vi "rsidr_core_global.vi"() -> ()   [LabVIEW 2020, in "Rohde&Schwarz RTx Oscilloscopes.lvlib"] (continued)
Options"="", "Flags"=0, "Help"="Queries the digital probe state.\n\nAvailable Repeated Capabilities:\nDigital: D0, D1, D2, D3, D4, D5, D6, D7, D8, D9, D10, D11, D12, D13, D14, D15\r\n\nRemote-control command(s):\nDIGital<m>:PROBe:ENABle?"}, {"Level"=2, "Class Only"=FALSE, "Identifier"="RSRTX_ATTR_DIGITAL_POINT_SELECTION", "Descriptive Name"="Digital Point Selection", "Data Type"=0, "Command"="DIG{Digital}:DATA:POIN", "Access"=1, "Range Table"="RsRtx_rngPointSelection", "Read Callback"="", "Write Callback"="", "Supported Models"="", "Instrument Options"="", "Flags"=0, "Help"="Selects a range of samples that will be returned. Depending on the current settings, the memory can contain more data samples than the screen is able to display. In this case, you can decide which data will be saved: samples stored in the memory or only the displayed samples.\n\nAvailable Repeated Capabilities:\nDigital: D0, D1, D2, D3, D4, D5, D6, D7, D8, D9, D10, D11, D12, D13, D14, D15\r\n\nRemote-control command(s):\nDIGital<m>:DATA:POINts"}, {"Level"=1, "Class Only"=TRUE, "Identifier"="", "Descriptive Name"="Logic", "Data Type"=0, "Command"="", "Access"=0, "Range Table"="", "Read Callback"="", "Write Callback"="", "Supported Models"="", "Instrument Options"="", "Flags"=0, "Help"="Configures the logic probe."}, {"Level"=2, "Class Only"=FALSE, "Identifier"="RSRTX_ATTR_LOGIC_STATE", "Descriptive Name"="Logic State", "Data Type"=3, "Command"="LOG{Logic}:STAT", "Access"=2, "Range Table"="", "Read Callback"="", "Write Callback"="", "Supported Models"="", "Instrument Options"="", "Flags"=0, "Help"="Enables the logic probe.\n\nAvailable Repeated Capabilities:\nLogic: Logic1, Logic2\r\n\nRemote-control command(s):\nLOGic<p>:STATe"}, {"Level"=2, "Class Only"=FALSE, "Identifier"="RSRTX_ATTR_LOGIC_TYPE", "Descriptive Name"="Logic Type", "Data Type"=0, "Command"="LOG{Logic}:TYPE", "Access"=2, "Range Table"="RsRtx_rngLogicType", "Read Callback"="", "Write Callback"="", "Supported Models"="", "Instrument Options"="", "Flags"=0, "Help"="Selects the logic type.\n\nAvailable Repeated Capabilities:\nLogic: Logic1, Logic2\r\n\nRemote-control command(s):\nLOGic<p>:TYPE"}, {"Level"=2, "Class Only"=FALSE, "Identifier"="RSRTX_ATTR_LOGIC_THRESHOLD", "Descriptive Name"="Logic Threshold", "Data Type"=0, "Command"="LOG{Logic}:THR", "Access"=2, "Range Table"="RsRtx_rngLogicThreshold", "Read Callback"="", "Write Callback"="", "Supported Models"="", "Instrument Options"="", "Flags"=0, "Help"="Configures logic threshold.\n\nAvailable Repeated Capabilities:\nLogic: Logic1, Logic2\r\n\nRemote-control command(s):\nLOGic<p>:THReshold"}, {"Level"=2, "Class Only"=FALSE, "Identifier"="RSRTX_ATTR_LOGIC_THRESHOLD_USER_LEVEL", "Descriptive Name"="Logic Threshold User Level", "Data Type"=1, "Command"="LOG{Logic}:THR:UDL", "Access"=2, "Range Table"="", "Read Callback"="", "Write Callback"="", "Supported Models"="", "Instrument Options"="", "Flags"=0, "Help"="Configures threshold user level.\n\nAvailable Repeated Capabilities:\nLogic: Logic1, Logic2\r\n\nRemote-control command(s):\nLOGic<p>:THReshold:UDLevel"}, {"Level"=2, "Class Only"=FALSE, "Identifier"="RSRTX_ATTR_LOGIC_HYSTERESIS", "Descriptive Name"="Logic Hysteresis", "Data Type"=0, "Command"="LOG{Logic}:HYST", "Access"=2, "Range Table"="rsrtx_rngLogicHysteresis", "Read Callback"="", "Write Callback"="", "Supported Models"="", "Instrument Options"="", "Flags"=0, "Help"="Configures logic hysteresis.\n\nAvailable Repeated Capabilities:\nLogic: Logic1, Logic2\r\n\nRemote-control command(s):\nLOGic<p>:HYSTeresis"}, {"Level"=2, "Class Only"=FALSE, "Identifier"="RSRTX_ATTR_LOGIC_ARITHMETICS", "Descriptive Name"="Logic Arithmetics", "Data Type"=0, "Command"="LOG{Logic}:ARIT", "Access"=2, "Range Table"="rsrtx_rngWaveformArithmetics", "Read Callback"="", "Write Callback"="", "Supported Models"="", "Instrument Options"="", "Flags"=0, "Help"="Configures logic arithmetics.\n\nAvailable Repeated Capabilities:\nLogic: Logic1, Logic2\r\n\nRemote-control command(s):\nLOGic<p>:ARIThmetics"}, {"Level"=2, "Class Only"=FALSE, "Identifier"="RSRTX_ATTR_LOGIC_PROBE_CONNECTED", "Descriptive Name"="Logic Probe Connected", "Data Type"=3, "Command"="LOG{Logic}:PROB?", "Access"=0, "Range Table"="", "Read Callback"="", "Write Callback"="", "Supported Models"="", "Instrument Options"="", "Flags"=0, "Help"="Checks if the logic probe is connected.\n\nAvailable Repeated Capabilities:\nLogic: Logic1, Logic2\r\n\nRemote-control command(s):\nLOGic<p>:PROBe[:ENABle]?"}, {"Level"=2, "Class Only"=FALSE, "Identifier"="RSRTX_ATTR_LOGIC_CURRENT_MAXIMUM", "Descriptive Name"="Logic Current Maximum", "Data Type"=0, "Command"="LOG{Logic}:CURR:STAT:MAX?", "Access"=0, "Range Table"="RsRtx_rngLogicCurrent", "Read Callback"="", "Write Callback"="", "Supported Models"="", "Instrument Options"="", "Flags"=0, "Help"="Queries current maximum.\n\nAvailable Repeated Capabilities:\nLogic: Logic1, Logic2\r\n\nRemote-control command(s):\nLOGic<p>:CURRent:STATe:MAXimum?"}, {"Level"=2, "Class Only"=FALSE, "Identifier"="RSRTX_ATTR_LOGIC_CURRENT_MINIMUM", "Descriptive Name"="Logic Current Minimum", "Data Type"=0, "Command"="LOG{Logic}:CURR:STAT:MIN?", "Access"=0, "Range Table"="RsRtx_rngLogicCurrent", "Read Callback"="", "Write Callback"="", "Supported Models"="", "Instrument Options"="", "Flags"=0, "Help"="Queries current minimum.\n\nAvailable Repeated Capabilities:\nLogic: Logic1, Logic2\r\n\nRemote-control command(s):\nLOGic<p>:CURRent:STATe:MINimum?"}, {"Level"=2, "Class Only"=FALSE, "Identifier"="RSRTX_ATTR_LOGIC_POINT_SELECTION", "Descriptive Name"="Logic Point Selection", "Data Type"=0, "Command"="LOG{Logic}:DATA:POIN", "Access"=1, "Range Table"="RsRtx_rngPointSelection", "Read Callback"="", "Write Callback"="", "Supported Models"="", "Instrument Options"="", "Flags"=0, "Help"="Selects a range of samples that will be returned with LOGic<p>:DATA. Depending on the current settings, the memory can contain more data samples than the screen is able to display. In this case, you can decide which data will be saved: samples stored in the memory or only the displayed samples.\n\nNote: The sample range can be changed only in STOP mode. If the acquisition is running, DEF is always used automatically. If the acquisition has been stopped, data can be read from the memory, and all settings are available.\n\nAvailable Repeated Capabilities:\nLogic: Logic1, Logic2\r\n\nRemote-control command(s):\nLOGic<p>:DATA:POINts"}, {"Level"=2, "Class Only"=FALSE, "Identifier"="RSRTX_ATTR_LOGIC_WAVEFORM_DATA_POINTS", "Descriptive Name"="Logic Waveform Data Points", "Data Type"=0, "Command"="LOG{Logic}:DATA:POIN?", "Access"=0, "Range Table"="", "Read Callback"="", "Write Callback"="", "Supported Models"="", "Instrument Options"="", "Flags"=0, "Help"="Returns the number of returned samples for the selected range.\n\nAvailable Repeated Capabilities:\nLogic: Logic1, Logic2\r\n\nRemote-control command(s):\nLOGic<p>:DATA:POINts?"}, {"Level"=1, "Class Only"=TRUE, "Identifier"="", "Descriptive Name"="Triggering Subsystem", "Data Type"=0, "Command"="", "Access"=0, "Range Table"="", "Read Callback"="", "Write Callback"="", "Supported Models"="", "Instrument Options"="", "Flags"=0, "Help"="Attributes that control how the oscilloscope triggers."}, {"Level"=2, "Class Only"=FALSE, "Identifier"="RSRTX_ATTR_TRIGGER_TYPE_A", "Descriptive Name"="Trigger Type A", "Data Type"=0, "Command"="TRIG:A:TYPE", "Access"=2, "Range Table"="rsrtx_rngTriggerType", "Read Callback"="", "Write Callback"="", "Supported Models"="", "Instrument Options"="", "Flags"=0, "Help"="Sets the trigger type.\n\nAvailable Repeated Capabilities:\nNone\n\nRemote-control command(s):\nTRIGger:A:TYPE"}, {"Level"=2, "Class Only"=FALSE, "Identifier"="RSRTX_ATTR_TRIGGER_SOURCE_A", "Descriptive Name"="Trigger Source A", "Data Type"=0, "Command"="TRIG:A:SOUR", "Access"=2, "Range Table"="rsrtx_rngTriggerSource", "Read Callback"="", "Write Callback"="", "Supported Models"="", "Instrument Options"="", "Flags"=0, "Help"="Sets the trigger source for the selected trigger type.\n\nAvailable Repeated Capabilities:\nNone\n\nRemote-control command(s):\nTRIGger:A:SOURce"}, {"Level"=2, "Class Only"=FALSE, "Identifier"="RSRTX_ATTR_TRIGGER_SOURCE_B", "Descriptive Name"="Trigger Source B", "Data Type"=0, "Command"="TRIG:B:SOUR", "Access"=2, "Range Table"="rsrtx_rngTriggerSource", "Read Callback"="", "Write Callback"="", "Supported Models"="", "Instrument Options"="", "Flags"=0, "Help"="Sets the trigger source for the selected trigger type.\n\nAvailable Repeated Capabilities:\nNone\n\nRemote-control command(s):\nTRIGger:B:SOURce"}, {"Level"=2, "Class Only"=FALSE, "Identifier"="RSRTX_ATTR_EXTERNAL_TRIGGER_COUPLING", "Descriptive Name"="External Trigger Coupling", "Data Type"=0, "Command"="TRIG:EXT:COUP", "Access"=2, "Range Table"="rsrtx_rngExternalTriggerCoupling", "Read Callback"="", "Write Callback"="", "Supported Models"="", "Instrument Options"="", "Flags"=0, "Help"="Sets the coupling for the external trigger input.\n\nAvailable Repeated Capabilities:\nNone\n\nRemote-control command(s):\nTRIGger:EXTern:COUPling"}, {"Level"=2, "Class Only"=FALSE, "Identifier"="RSRTX_ATTR_EXTERNAL_TRIGGER_TERMINATION", "Descriptive Name"="External Trigger Termination", "Data Type"=3, "Command"="TRIG:EXT:TERM", "Access"=2, "Range Table"="", "Read Callback"="", "Write Callback"="", "Supported Models"="", "Instrument Options"="", "Flags"=0, "Help"="Adjusts the input impedance of the external trigger input.\nOnly available for instruments with 1 GHz bandwidth.\n\nAvailable Repeated Capabilities:\nNone\n\nRemote-control command(s):\nTRIGger:EXTern:TERMination"}, {"Level"=2, "Class Only"=FALSE, "Identifier"="RSRTX_ATTR_EXTERNAL_TRIGGER_OVERLOAD", "Descriptive Name"="External Trigger Overload", "Data Type"=3, "Command"="TRIG:EXT:OVER", "Access"=2, "Range Table"="", "Read Callback"="", "Write Callback"="", "Supported Models"="", "Instrument Options"="", "Flags"=0, "Help"="Retrieves the overload status of the external trigger input from the status bit. When the overload problem is solved, use the command to reset the status bit.\nOnly available for instruments with 1 GHz bandwidth.\n\nAvailable Repeated Capabilities:\nNone\n\nRemote-control command(s):\nTRIGger:EXTern:OVERload"}, {"Level"=2, "Class Only"=FALSE, "Identifier"="RSRTX_ATTR_TRIGGER_HOLDOFF_TIME", "Descriptive Name"="Trigger Holdoff Time", "Data Type"=1, "Command"="TRIG:A:HOLD:TIME", "Access"=2, "Range Table"="", "Read Callback"="", "Write Callback"="", "Supported Models"="", "Instrument Options"="", "Flags"=0, "Help"="Defines the holdoff time. The next trigger occurs only after the holdoff time has passed.\n\nAvailable Repeated Capabilities:\nNone\n\nRemote-control command(s):\nTRIGger:A:HOLDoff:TIME"}, {"Level"=2, "Class Only"=FALSE, "Identifier"="RSRTX_ATTR_TRIGGER_HOLDOFF_MODE", "Descriptive Name"="Trigger Holdoff Mode", "Data Type"=0, "Command"="TRIG:A:HOLD:MODE", "Access"=2, "Range Table"="rsrtx_rngTriggerHoldoffMode", "Read Callback"="", "Write Callback"="", "Supported Models"="", "Instrument Options"="", "Flags"=0, "Help"="Enables or disables the holdoff time.\n\nAvailable Repeated Capabilities:\nNone\n\nRemote-control command(s):\nTRIGger:A:HOLDoff:MODE"}, {"Level"=2, "Class Only"=FALSE, "Identifier"="RSRTX_ATTR_TRIGGER_HYSTERESIS_A", "Descriptive Name"="Trigger Hysteresis A", "Data Type"=0, "Command"="TRIG:A:HYST", "Access"=2, "Range Table"="rsrtx_rngHysteresisMode", "Read Callback"="", "Write Callback"="", "Supported Models"="", "Instrument Options"="", "Flags"=0, "Help"="Sets a hysteresis range around the trigger level of the A trigger event. If the signal jitters inside this range and crosses the trigger level thereby, no trigger event occurs. Hysteresis is available for edge and width trigger.\n\nAvailable Repeated Capabilities:\nNone\n\nRemote-control command(s):\nTRIGger:A:HYSTeresis"}, {"Level"=2, "Class Only"=FALSE, "Identifier"="RSRTX_ATTR_TRIGGER_HYSTERESIS_A_LEVEL", "Descriptive Name"="Trigger Hysteresis A Level", "Data Type"=0, "Command"="TRIG:A:LEV1:HYST", "Access"=2, "Range Table"="", "Read Callback"="", "Write Callback"="", "Supported Models"="RTM|RTA", "Instrument Options"="", "Flags"=0, "Help"="Sets the hysteresis value if TRIGger:A:HYSTeresis is set to MANual. Only available on instruments with 1 GHz bandwidth.\n\nAvailable Repeated Capabilities:\nNone\n\nRemote-control command(s):\nTRIGger:A:LEVel<n>:HYSTeresis"}, {"Level"=2, "Class Only"=FALSE, "Identifier"="RSRTX_ATTR_TRIGGER_HYSTERESIS_B", "Descriptive Name"="Trigger Hysteresis B", "Data Type"=0, "Command"="TRIG:B:HYST", "Access"=2, "Range Table"="rsrtx_rngHysteresisMode", "Read Callback"="", "Write Callback"="", "Supported Models"="", "Instrument Options"="", "Flags"=0, "Help"="Sets a hysteresis range around the trigger level of the A trigger event. If the signal jitters inside this range and crosses the trigger level thereby, no trigger event occurs. Hysteresis is available for edge and width trigger.\n\nAvailable Repeated Capabilities:\nNone\n\nRemote-control command(s):\nTRIGger:B:HYSTeresis"}, {"Level"=2, "Class Only"=FALSE, "Identifier"="RSRTX_ATTR_TRIGGER_HYSTERESIS_B_LEVEL", "Descriptive Name"="Trigger Hysteresis B Level", "Data Type"=0, "Command"="TRIG:B:LEV:HYST", "Access"=2, "Range Table"="", "Read Callback"="", "Write Callback"="", "Supported Models"="", "Instrument Options"="", "Flags"=0, "Help"="Sets the hysteresis value if TRIGger:B:HYSTeresis is set to MANual. Only available on instruments with 1 GHz bandwidth.\n\nAvailable Repeated Capabilities:\nNone\n\nRemote-control command(s):\nTRIGger:B:LEVel:HYSTeresis"}, {"Level"=2, "Class Only"=FALSE, "Identifier"="RSRTX_ATTR_TRIGGER_ENABLED", "Descriptive Name"="Trigger Enabled", "Data Type"=3, "Command"="TRIG:B:ENAB", "Access"=2, "Range Table"="", "Read Callback"="", "Write Callback"="", "Supported Models"="", "Instrument Options"="", "Flags"=0, "Help"="Activates or deactivates the second trigger. The instrument triggers if both trigger event conditions (A and B) are fulfilled.\n\nAvailable Repeated Capabilities:\nNone\n\nRemote-control command(s):\nTRIGger:B:ENABle"}, {"Level"=2, "Class Only"=FALSE, "Identifier"="RSRTX_ATTR_TRIGGER_MODIFIER_A", "Descriptive Name"="Trigger Modifier A", "Data Type"=0, "Command"="TRIG:A:MODE", "Access"=2, "Range Table"="rsrtx_rngTriggerMode", "Read Callback"="", "Write Callback"="", "Supported Models"="", "Instrument Options"="", "Flags"=0, "Help"="Sets the trigger mode. The trigger mode determines the behaviour of the instrument if no trigger occurs.\n\nAvailable Repeated Capabilities:\nNone\n\nRemote-control command(s):\nTRIGger:A:MODE"}, {"Level"=2, "Class Only"=FALSE, "Identifier"="RSRTX_ATTR_TRIGGER_MODIFIER_B", "Descriptive Name"="Trigger Modifier B", "Data Type"=0, "Command"="TRIG:B:MODE", "Access"=2, "Range Table"="rsrtx_rngTriggerMode", "Read Callback"="", "Write Callback"="", "Supported Models"="", "Instrument Options"="", "Flags"=0, "Help"="Sets the trigger mode. The trigger mode determines the behaviour of the instrument if no trigger occurs.\n\nAvailable Repeated Capabilities:\nNone\n\nRemote-control command(s):\nTRIGger:B:MODE"}, {"Level"=2, "Class Only"=FALSE, "Identifier"="RSRTX_ATTR_TRIGGER_EVENT_COUNT", "Descriptive Name"="Trigger Event Count", "Data Type"=0, "Command"="TRIG:B:EVEN:COUN", "Access"=2, "Range Table"="", "Read Callback"="", "Write Callback"="", "Supported Models"="", "Instrument Options"="", "Flags"=0, "Help"="Sets a number of B-trigger events that fulfill all B-trigger conditions but do not cause the trigger. The oscilloscope triggers on the n-th event (the last of the specified number of events).\n\nAvailable Repeated Capabilities:\nNone\n\nRemote-control command(s):\nTRIGger:B:EVENt:COUNt"}, {"Level"=2, "Class Only"=FALSE, "Identifier"="RSRTX_ATTR_TRIGGER_LEVEL_AUTO_FIND_A", "Descriptive Name"="Trigger Level Auto Find A", "Data Type"=4, "Command"="TRIG:A:FIND", "Access"=1, "Range Table"="", "Read Callback"="", "Write Callback"="", "Supported Models"="", "Instrument Options"="", "Flags"=0, "Help"="Sets the trigger level automatically. Not available for an external trigger source.\n\nAvailable Repeated Capabilities:\nNone\n\nRemote-control command(s):\nTRIGger:A:FINDlevel"}, {"Level"=2, "Class Only"=FALSE, "Identifier"="RSRTX_ATTR_TRIGGER_LEVEL_AUTO_FIND_B", "Descriptive Name"="Trigger Level Auto Find B", "Data Type"=4, "Command"="TRIG:B:FIND", "Access"=1, "Range Table"="", "Read Callback"="", "Write Callback"="", "Supported Models"="", "Instrument Options"="", "Flags"=0, "Help"="Sets the trigger level automatically. Not available for an external trigger source.\n\nAvailable Repeated Capabilities:\nNone\n\nRemote-control command(s):\nTRIGger:B:FINDlevel"}, {"Level"=2, "Class Only"=FALSE, "Identifier"="RSRTX_ATTR_TRIGGER_LEVEL_LOWER", "Descriptive Name"="Trigger Level Lower", "Data Type"=1, "Command"="TRIG:A:LEV1:RIS:LOW", "Access"=2, "Range Table"="", "Read Callback"="", "Write Callback"="", "Supported Models"="RTM|RTA", "Instrument Options"="", "Flags"=0, "Help"="Set the lower voltage threshold, respectively. When the signal crosses these levels, the slew rate measurement starts or stops depending on the selected polarity.\n\nAvailable Repeated Capabilities:\nNone\n\nRemote-control command(s):\nTRIGger:A:LEVel<n>:RISetime:LOWer"}, {"Level"=2, "Class Only"=FALSE, "Identifier"="RSRTX_ATTR_TRIGGER_LEVEL_UPPER", "Descriptive Name"="Trigger Level Upper", "Data Type"=1, "Command"="TRIG:A:LEV1:RIS:UPP", "Access"=2, "Range Table"="", "Read Callback"="", "Write Callback"="", "Supported Models"="RTM|RTA", "Instrument Options"="", "Flags"=0, "Help"="Set the uper voltage threshold, respectively. When the signal crosses these levels, the slew rate measurement starts or stops depending on the selected polarity.\n\nAvailable Repeated Capabilities:\nNone\n\nRemote-control command(s):\nTRIGger:A:LEVel<n>:RISetime:UPPer"}, {"Level"=2, "Class Only"=FALSE, "Identifier"="RSRTX_ATTR_TRIGGER_DELAY", "Descriptive Name"="Trigger Delay", "Data Type"=1, "Command"="TRIG:B:DEL", "Access"=2, "Range Table"="rsrtx_rngTrgDelay", "Read Callback"="", "Write Callback"="", "Supported Models"="", "Instrument Options"="", "Flags"=0, "Help"="Sets the time the instrument waits after an A-event until it recognizes B-events. Before setting the dalay time, TRIGger: B: MODE must be set to DELAy.\n\nAvailable Repeated Capabilities:\nNone\n\nRemote-control command(s):\nTRIGger:B:DELay"}, {"Level"=2, "Class Only"=TRUE, "Identifier"="", "Descriptive Name"="Channel", "Data Type"=0, "Command"="", "Access"=0, "Range Table"="", "Read Callback"="", "Write Callback"="", "Supported Models"="", "Instrument Options"="", "Flags"=0, "Help"="Attributes that control how the oscilloscope triggers."}, {"Level"=3, "Class Only"=FALSE, "Identifier"="RSRTX_ATTR_TRIGGER_LEVEL_A", "Descriptive Name"="Trigger Level A", "Data Type"=1, "Command"="TRIG:A:LEV{Channel}", "Access"=2, "Range Table"="rsrtx_rngTriggerLevel", "Read Callback"="", "Write Callback"="", "Supported Models"="", "Instrument Options"="", "Flags"=0, "Help"="Sets the trigger level for the specified event and source.\n\nAvailable Repeated Capabilities:\nChannel: CH0, CH1, CH2, CH3, CH4, CHExt\r\n\nRemote-control command(s):\nTRIGger:A:LEVel<n>[:VALue]"}, {"Level"=3, "Class Only"=FALSE, "Identifier"="RSRTX_ATTR_TRIGGER_LEVEL_B", "Descriptive Name"="Trigger Level B", "Data Type"=1, "Command"="TRIG:B:LEV{Channel}", "Access"=2, "Range Table"="", "Read Callback"="", "Write Callback"="", "Supported Models"="", "Instrument Options"="", "Flags"=0, "Help"="Sets the trigger level for the specified event and source.\n\nAvailable Repeated Capabilities:\nChannel: CH0, CH1, CH2, CH3, CH4, CHExt\r\n\nRemote-control command(s):\nTRIGger:B:LEVel<n>[:VALue]"}, {"Level"=2, "Class Only"=TRUE, "Identifier"="", "Descriptive Name"="Edge Triggering", "Data Type"=0, "Command"="", "Access"=0, "Range Table"="", "Read Callback"="", "Write Callback"="", "Supported Models"="", "Instrument Options"="", "Flags"=0, "Help"="Attributes that configure the edge trigger.  An edge trigger occurs when the trigger signal passes through the voltage threshold you specify with the RSRTX_ATTR_TRIGGER_LEVEL attribute and has the slope you specify with the RSRTX_ATTR_TRIGGER_SLOPE attribute."}, {"Level"=3, "Class Only"=FALSE, "Identifier"="RSRTX_ATTR_TRIGGER_SLOPE_A", "Descriptive Name"="Trigger Slope A", "Data Type"=0, "Command"="TRIG:A:EDGE:SLOP", "Access"=2, "Range Table"="rsrtx_rngTriggerSlope", "Read Callback"="", "Write Callback"="", "Supported Models"="", "Instrument Options"="", "Flags"=0, "Help"="Sets the slope for the edge trigger.\n\nAvailable Repeated Capabilities:\nNone\n\nRemote-control command(s):\nTRIGger:A:EDGE:SLOPe"}, {"Level"=3, "Class Only"=FALSE, "Identifier"="RSRTX_ATTR_TRIGGER_SLOPE_B", "Descriptive Name"="Trigger Slope B", "Data Type"=0, "Command"="TRIG:B:EDGE:SLOP", "Access"=2, "Range Table"="rsrtx_rngTriggerSlope", "Read Callback"="", "Write Callback"="", "Supported Models"="", "Instrument Options"="", "Flags"=0, "Help"="Sets the slope for the edge trigger.\n\nAvailable Repeated Capabilities:\nNone\n\nRemote-control command(s):\nTRIGger:B:EDGE:SLOPe"}, {"Level"=3, "Class Only"=FALSE, "Identifier"="RSRTX_ATTR_TRIGGER_COUPLING", "Descriptive Name"="Trigger Coupling", "Data Type"=0, "Command"="TRIG:A:EDGE:COUP", "Access"=2, "Range Table"="rsrtx_rngTriggerCoupling", "Read Callback"="", "Write Callback"="", "Supported Models"="", "Instrument Options"="", "Flags"=0, "Help"="Sets the coupling for the trigger source.\n\nAvailable Repeated Capabilities:\nNone\n\nRemote-control command(s):\nTRIGger:A:EDGE:COUPling"}, {"Level"=3, "Class Only"=FALSE, "Identifier"="RSRTX_ATTR_TRIGGER_FILTER_HIGH", "Descriptive Name"="Trigger Filter High", "Data Type"=3, "Command"="TRIG:A:EDGE:FILT:NREJ", "Access"=2, "Range Table"="", "Read Callback"="", "Write Callback"="", "Supported Models"="", "Instrument Options"="", "Flags"=0, "Help"="Turns an additional high-pass filter in the trigger path on or off. This filter removes higher frequencies and is available with AC and DC coupling.\n\nAvailable Repeated Capabilities:\nNone\n\nRemote-control command(s):\nTRIGger:A:EDGE:FILTer:NREJect"}, {"Level"=3, "Class Only"=FALSE, "Identifier"="RSRTX_ATTR_TRIGGER_FILTER_HF_REJECT", "Descriptive Name"="Trigger Filter HF Reject", "Data Type"=3, "Command"="TRIG:A:EDGE:FILT:HFR", "Access"=2, "Range Table"="", "Read Callback"="", "Write Callback"="", "Supported Models"="", "Instrument Options"="", "Flags"=0, "Help"="Enables or disables an additional 5 kHz lowpass filter in the trigger path. This filter removes higher frequencies and is available with AC and DC coupling.\n\nAvailable Repeated Capabilities:\nNone\n\nRemote-control command(s):\nTRIGger:A:EDGE:FILTer:HFReject"}, {"Level"=2, "Class Only"=TRUE, "Identifier"="", "Descriptive Name"="TV Triggering", "Data Type"=0, "Command"="", "Access"=0, "Range Table"="", "Read Callback"="", "Write Callback"="", "Supported Models"="", "Instrument Options"="", "Flags"=0, "Help"="Attributes that configure the oscilloscope to trigger on TV signals."}, {"Level"=3, "Class Only"=FALSE, "Identifier"="RSRTX_ATTR_TV_TRIGGER_EVENT", "Descriptive Name"="TV Trigger Event", "Data Type"=0, "Command"="TRIG:A:TV:FIEL", "Access"=2, "Range Table"="rsrtx_rngTVTriggerEvent", "Read Callback"="", "Write Callback"="", "Supported Models"="", "Instrument Options"="", "Flags"=0, "Help"="Sets the trigger on the beginning of the video signal fields, or on the beginning of video signal lines.\n\nAvailable Repeated Capabilities:\nNone\n\nRemote-control command(s):\nTRIGger:A:TV:FIELd"}, {"Level"=3, "Class Only"=FALSE, "Identifier"="RSRTX_ATTR_TV_TRIGGER_LINE_NUMBER", "Descriptive Name"="TV Trigger Line Number", "Data Type"=0, "Command"="TRIG:A:TV:LINE", "Access"=2, "Range Table"="rsrtx_rngLineNumber", "Read Callback"="", "Write Callback"="", "Supported Models"="", "Instrument Options"="", "Flags"=0, "Help"="Sets an exact line number if Trigger Event is set to LINE.\n\nAvailable Repeated Capabilities:\nNone\n\nRemote-control command(s):\nTRIGger:A:TV:LINE"}, {"Level"=3, "Class Only"=FALSE, "Identifier"="RSRTX_ATTR_TV_TRIGGER_POLARITY", "Descriptive Name"="TV Trigger Polarity", "Data Type"=0, "Command"="TRIG:A:TV:POL", "Access"=2, "Range Table"="rsrtx_rngPolarity", "Read Callback"="", "Write Callback"="", "Supported Models"="", "Instrument Options"="", "Flags"=0, "Help"="Sets the polarity of the sync pulses. The edges of the sync pulses are used for triggering.\n\nAvailable Repeated Capabilities:\nNone\n\nRemote-control command(s):\nTRIGger:A:TV:POLarity"}, {"Level"=3, "Class Only"=FALSE, "Identifier"="RSRTX_ATTR_TV_STANDARD", "Descriptive Name"="TV Standard", "Data Type"=0, "Command"="TRIG:A:TV:STAN", "Access"=2, "Range Table"="rsrtx_rngTVStandard", "Read Callback"="", "Write Callback"="", "Supported Models"="", "Instrument Options"="", "Flags"=0, "Help"="Selects the color television standard.\n\nAvailable Repeated Capabilities:\nNone\n\nRemote-control command(s):\nTRIGger:A:TV:STANdard"}, {"Level"=2, "Class Only"=TRUE, "Identifier"="", "Descriptive Name"="Width Triggering", "Data Type"=0, "Command"="", "Access"=0, "Range Table"="", "Read Callback"="", "Write Callback"="", "Supported Models"="", "Instrument Options"="", "Flags"=0, "Help"="Width Triggering"}, {"Level"=3, "Class Only"=FALSE, "Identifier"="RSRTX_ATTR_WIDTH", "Descriptive Name"="Width", "Data Type"=1, "Command"="TRIG:A:WIDT:WIDT", "Access"=2, "Range Table"="", "Read Callback"="", "Write Callback"="", "Supported Models"="", "Instrument Options"="", "Flags"=0, "Help"="For the ranges WITHin and OUTSide, the <Time1> defines the center of a range which is defined by the limits +-<Delta>. For the ranges SHORter and LONGer, the width defines the maximum and minimum pulse width, respectively.\n\nAvailable Repeated Capabilities:\nNone\n\nRemote-control command(s):\nTRIGger:A:WIDTh:WIDTh"}, {"Level"=3, "Class Only"=FALSE, "Identifier"="RSRTX_ATTR_WIDTH_DELTA", "Descriptive Name"="Width Delta", "Data Type"=1, "Command"="TRIG:A:WIDT:DELT", "Access"=2, "Range Table"="", "Read Callback"="", "Write Callback"="", "Supported Models"="", "Instrument Options"="", "Flags"=0, "Help"="Defines a range around the width value.\n\nAvailable Repeated Capabilities:\nNone\n\nRemote-control command(s):\nTRIGger:A:WIDTh:DELTa"}, {"Level"=3, "Class Only"=FALSE, "Identifier"="RSRTX_ATTR_WIDTH_POLARITY", "Descriptive Name"="Width Polarity", "Data Type"=0, "Command"="TRIG:A:WIDT:POL", "Access"=2, "Range Table"="rsrtx_rngPolarity", "Read Callback"="", "Write Callback"="", "Supported Models"="", "Instrument Options"="", "Flags"=0, "Help"="Sets the polarity of the pulse.\n\nAvailable Repeated Capabilities:\nNone\n\nRemote-control command(s):\nTRIGger:A:WIDTh:POLarity"}, {"Level"=3, "Class Only"=FALSE, "Identifier"="RSRTX_ATTR_WIDTH_CONDITION", "Descriptive Name"="Width Condition", "Data Type"=0, "Command"="TRIG:A:WIDT:RANG", "Access"=2, "Range Table"="rsrtx_rngWidthCondition", "Read Callback"="", "Write Callback"="", "Supported Models"="", "Instrument Options"="", "Flags"=0, "Help"="Defines how the measured pulse width is compared with the given limit(s).\n\nAvailable Repeated Capabilities:\nNone\n\nRemote-control command(s):\nTRIGger:A:WIDTh:RANGe"}, {"Level"=2, "Class Only"=TRUE, "Identifier"="", "Descriptive Name"="Trigger Pattern", "Data Type"=0, "Command"="", "Access"=0, "Range Table"="", "Read Callback"="", "Write Callback"="", "Supported Models"="", "Instrument Options"="", "Flags"=0, "Help"="Atributes configures the Pattern Trigger."}, {"Level"=3, "Class Only"=FALSE, "Identifier"="RSRTX_ATTR_TRIGGER_PATTERN_SOURCE", "Descriptive Name"="Trigger Pattern Source", "Data Type"=2, "Command"="TRIG:A:PATT:SOUR", "Access"=2, "Range Table"="", "Read Callback"="", "Write Callback"="", "Supported Models"="", "Instrument Options"="", "Flags"=0, "Help"="Select the state for each digital channel.\n\nAvailable Repeated Capabilities:\nNone\n\nRemote-control command(s):\nTRIGger:A:PATTern:SOURce"}, {"Level"=3, "Class Only"=FALSE, "Identifier"="RSRTX_ATTR_TRIGGER_PATTERN_FUNCTION", "Descriptive Name"="Trigger Pattern Function", "Data Type"=0, "Command"="TRIG:A:PATT:FUNC", "Access"=2, "Range Table"="rsrtx_rngTriggerPatternFunction", "Read Callback"="", "Write Callback"="", "Supported Models"="", "Instrument Options"="", "Flags"=0, "Help"="Sets the logical combination of the trigger states of the channels.\n\nAvailable Repeated Capabilities:\nNone\n\nRemote-control command(s):\nTRIGger:A:PATTern:FUNCtion"}, {"Level"=3, "Class Only"=FALSE, "Identifier"="RSRTX_ATTR_TRIGGER_PATTERN_POINT_ENABLED", "Descriptive Name"="Trigger Pattern Point Enabled", "Data Type"=3, "Command"="TRIG:A:PATT:COND", "Access"=2, "Range Table"="", "Read Callback"="rsrtx_PatternCondition_ReadCallback.vi", "Write Callback"="rsrtx_PatternCondition_WriteCallback.vi", "Supported Models"="", "Instrument Options"="", "Flags"=0, "Help"="Sets the trigger point depending on the result of the logical combination of the channel states.\n\nAvailable Repeated Capabilities:\nNone\n\nRemote-control command(s):\nTRIGger:A:PATTern:CONDition"}, {"Level"=3, "Class Only"=FALSE, "Identifier"="RSRTX_ATTR_TRIGGER_PATTERN_MODE", "Descriptive Name"="Trigger Pattern Mode", "Data Type"=0, "Command"="TRIG:A:PATT:MODE", "Access"=2, "Range Table"="rsrtx_rngTriggerPatternMode", "Read Callback"="", "Write Callback"="", "Supported Models"="", "Instrument Options"="", "Flags"=0, "Help"="Disables the time limitation or sets the time comparison mode.\n\nAvailable Repeated Capabilities:\nNone\n\nRemote-control command(s):\nTRIGger:A:PATTern:MODE"}, {"Level"=3, "Class Only"=FALSE, "Identifier"="RSRTX_ATTR_TRIGGER_PATTERN_WIDTH", "Descriptive Name"="Trigger Pattern Width", "Data Type"=1, "Command"="TRIG:A:PATT:WIDT", "Access"=2, "Range Table"="", "Read Callback"="", "Write Callback"="", "Supported Models"="", "Instrument Options"="", "Flags"=0, "Help"="For the ranges WITHin and OUTSide, the <PatternWidth> defines the center of a range which is defined by the limits <Delta>.\n\nFor the ranges SHORter and LONGer, the pattern width defines the maximum and minimum values, respectively.\n\nAvailable Repeated Capabilities:\nNone\n\nRemote-control command(s):\nTRIGger:A:PATTern:WIDTh[:WIDTh]"}, {"Level"=3, "Class Only"=FALSE, "Identifier"="RSRTX_ATTR_TRIGGER_PATTERN_WIDTH_DELTA", "Descriptive Name"="Trigger Pattern Width Delta", "Data Type"=1, "Command"="TRIG:A:PATT:WIDT:DELT", "Access"=2, "Range Table"="", "Read Callback"="", "Write Callback"="", "Supported Models"="", "Instrument Options"="", "Flags"=0, "Help"="Defines a range around the pattern width value specified using TRIGger:A:PATTern:WIDTh[:WIDTh].\n\nAvailable Repeated Capabilities:\nNone\n\nRemote-control command(s):\nTRIGger:A:PATTern:WIDTh:DELTa"}, {"Level"=3, "Class Only"=FALSE, "Identifier"="RSRTX_ATTR_TRIGGER_PATTERN_WIDTH_CONDITION", "Descriptive Name"="Trigger Pattern Width Condition", "Data Type"=0, "Command"="TRIG:A:PATT:WIDT:RANG", "Access"=2, "Range Table"="rsrtx_rngWidthCondition", "Read Callback"="", "Write Callback"="", "Supported Models"="", "Instrument Options"="", "Flags"=0, "Help"="Selects how the time limit of the pattern state is defined.\n\nAvailable Repeated Capabilities:\nNone\n\nRemote-control command(s):\nTRIGger:A:PATTern:WIDTh:RANGe"}, {"Level"=2, "Class Only"=TRUE, "Identifier"="", "Descriptive Name"="Window", "Data Type"=0, "Command"="", "Access"=0, "Range Table"="", "Read Callback"="", "Write Callback"="", "Supported Models"="", "Instrument Options"="", "Flags"=0, "Help"="Window Triggering."}, {"Level"=3, "Class Only"=FALSE, "Identifier"="RSRTX_ATTR_TRIGGER_WINDOW_RANGE", "Descriptive Name"="Trigger Window Range", "Data Type"=0, "Command"="TRIG:A:WIND:RANG", "Access"=2, "Range Table"="rsrtx_rngWindowRange", "Read Callback"="", "Write Callback"="", "Supported Models"="RTM|RTA", "Instrument Options"="", "Flags"=0, "Help"="Sets how the measured pulse width is compared with the given limit(s).\n\nAvailable Repeated Capabilities:\nNone\n\nRemote-control command(s):\nTRIGger:A:WINDow:RANGe"}, {"Level"=3, "Class Only"=FALSE, "Identifier"="RSRTX_ATTR_TRIGGER_WINDOW_WIDTH", "Descriptive Name"="Trigger Window Width", "Data Type"=1, "Command"="TRIG:A:WIND:WIDT", "Access"=2, "Range Table"="", "Read Callback"="", "Write Callback"="", "Supported Models"="RTM|RTA", "Instrument Options"="", "Flags"=0, "Help"="Configures window trigger width.\n\nAvailable Repeated Capabilities:\nNone\n\nRemote-control command(s):\nTRIGger:A:WINDow:WIDTh"}, {"Level"=3, "Class Only"=FALSE, "Identifier"="RSRTX_ATTR_TRIGGER_WINDOW_TIME_RANGE", "Descriptive Name"="Trigger Window Time Range", "Data Type"=0, "Command"="TRIG:A:WIND:TIME", "Access"=2, "Range Table"="rsrtx_rngWidthCondition", "Read Callback"="", "Write Callback"="", "Supported Models"="RTM|RTA", "Instrument Options"="", "Flags"=0, "Help"="Configures the window time range.\n\nAvailable Repeated Capabilities:\nNone\n\nRemote-control command(s):\nTRIGger:A:WINDow:TIME"}, {"Level"=2, "Class Only"=TRUE, "Identifier"="", "Descriptive Name"="Trigger Time", "Data Type"=0, "Command"="", "Access"=0, "Range Table"="", "Read Callback"="", "Write Callback"="", "Supported Models"="", "Instrument Options"="", "Flags"=0, "Help"="Atributes configures the Trigger Time."}, {"Level"=3, "Class Only"=FALSE, "Identifier"="RSRTX_ATTR_TRIGGER_TIME_POLARITY", "Descriptive Name"="Trigger Time Polarity", "Data Type"=0, "Command"="TRIG:A:RIS:SLOP", "Access"=2, "Range Table"="rsrtx_rngPolarity", "Read Callback"="", "Write Callback"="", "Supported Models"="RTM|RTA", "Instrument Options"="", "Flags"=0, "Help"="Sets the edge of whic the transition time is to be analyzed.\n\nAvailable Repeated Capabilities:\nNone\n\nRemote-control command(s):\nTRIGger:A:RISetime:SLOPe"}, {"Level"=3, "Class Only"=FALSE, "Identifier"="RSRTX_ATTR_TRIGGER_TIME_CONDITION", "Descriptive Name"="Trigger Time Condition", "Data Type"=0, "Command"="TRIG:A:RIS:RANG", "Access"=2, "Range Table"="rsrtx_rngWidthCondition", "Read Callback"="", "Write Callback"="", "Supported Models"="RTM|RTA", "Instrument Options"="", "Flags"=0, "Help"="Selects how the time limit of the rise or fall time is defined.\n\nAvailable Repeated Capabilities:\nNone\n\nRemote-control command(s):\nTRIGger:A:RISetime:RANGe"}, {"Level"=3, "Class Only"=FALSE, "Identifier"="RSRTX_ATTR_TRIGGER_TIME", "Descriptive Name"="Trigger Time", "Data Type"=1, "Command"="TRIG:A:RIS:TIME", "Access"=2, "Range Table"="", "Read Callback"="", "Write Callback"="", "Supported Models"="RTM|RTA", "Instrument Options"="", "Flags"=0, "Help"="For the ranges LONGer and SHORter, the command defines the minimum and maximum transition times, respectively.\n\nFor the ranges WITHin and OUTSide, the command defines the center of a time range which is defined using TRIGger:A:RISetime:DELTa.\n\nAvailable Repeated Capabilities:\nNone\n\nRemote-control command(s):\nTRIGger:A:RISetime:TIME"}, {"Level"=3, "Class Only"=FALSE, "Identifier"="RSRTX_ATTR_TRIGGER_TIME_DELTA", "Descriptive Name"="Trigger Time Delta", "Data Type"=1, "Command"="TRIG:A:RIS:DELT", "Access"=2, "Range Table"="", "Read Callback"="", "Write Callback"="", "Supported Models"="RTM|RTA", "Instrument Options"="", "Flags"=0, "Help"="Sets a time range around the time value defined using TRIGger:A:RISetime:TIME if TRIGger:A:RISetime:RANGe is set to WITHin | OUTSide.\n\nAvailable Repeated Capabilities:\nNone\n\nRemote-control command(s):\nTRIGger:A:RISetime:DELTa"}, {"Level"=2, "Class Only"=TRUE, "Identifier"="", "Descriptive Name"="Actions On Trigger", "Data Type"=0, "Command"="", "Access"=0, "Range Table"="", "Read Callback"="", "Write Callback"="", "Supported Models"="", "Instrument Options"="", "Flags"=0, "Help"="A trigger event can be used to initiate one or several actions. All available actions can be initiated at the same time, and for all trigger types."}, {"Level"=3, "Class Only"=FALSE, "Identifier"="RSRTX_ATTR_ACTIONS_ON_TRIGGER_ENABLED", "Descriptive Name"="Actions On Trigger Enabled", "Data Type"=3, "Command"="TRIG:EVEN", "Access"=2, "Range Table"="", "Read Callback"="", "Write Callback"="", "Supported Models"="", "Instrument Options"="", "Flags"=0, "Help"="Activates the selected actions on trigger event.\n\nAvailable Repeated Capabilities:\nNone\n\nRemote-control command(s):\nTRIGger:EVENt[:ENABle]"}, {"Level"=3, "Class Only"=FALSE, "Identifier"="RSRTX_ATTR_ACTIONS_ON_TRIGGER_SOUND", "Descriptive Name"="Actions On Trigger Sound", "Data Type"=3, "Command"="TRIG:EVEN:SOUN", "Access"=2, "Range Table"="", "Read Callback"="", "Write Callback"="", "Supported Models"="", "Instrument Options"="", "Flags"=0, "Help"="If ON, the instrument generates a beep on trigger event. The acquisition is not delayed, the sound generation runs asynchronously. The minimum time between two beeps is 1 s. If the instrument triggers faster, not all events are notified by a beep.\n\nAvailable Repeated Capabilities:\nNone\n\nRemote-control command(s):\nTRIGger:EVENt:SOUNd"}, {"Level"=3, "Class Only"=FALSE, "Identifier"="RSRTX_ATTR_ACTIONS_ON_TRIGGER_SCREENSHOT", "Descriptive Name"="Actions On Trigger Screenshot", "Data Type"=3, "Command"="TRIG:EVEN:SCRS", "Access"=2, "Range Table"="", "Read Callback"="", "Write Callback"="", "Supported Models"="", "Instrument Options"="", "Flags"=0, "Help"="If ON, the instrument saves a screenshot on each trigger event. The screenshot is saved when the acquisition is complete. During saving, the acquisition stops, and restarts when saving is finished. Thus, the waveform update rate decreases significantly.\n\nAvailable Repeated Capabilities:\nNone\n\nRemote-control command(s):\nTRIGger:EVENt:SCRSave"}, {"Level"=3, "Class Only"=FALSE, "Identifier"="RSRTX_ATTR_ACTIONS_ON_TRIGGER_SCREENSHOT_DESTINATION", "Descriptive Name"="Actions On Trigger Screenshot Destination", "Data Type"=2, "Command"="TRIG:EVEN:SCRS:DEST", "Access"=2, "Range Table"="", "Read Callback"="", "Write Callback"="", "Supported Models"="", "Instrument Options"="", "Flags"=0, "Help"="Defines the target directory and file name for a screenshot that is saved on trigger event when RSRTX_ATTR_ACTIONS_ON_TRIGGER_SCREENSHOT is ON.\n\nAvailable Repeated Capabilities:\nNone\n\nRemote-control command(s):\nTRIGger:EVENt:SCRSave:DESTination"}, {"Level"=3, "Class Only"=FALSE, "Identifier"="RSRTX_ATTR_ACTIONS_ON_TRIGGER_SAVE_WAVEFORM", "Descriptive Name"="Actions On Trigger Save Waveform", "Data Type"=3, "Command"="TRIG:EVEN:WFMS", "Access"=2, "Range Table"="", "Read Callback"="", "Write Callback"="", "Supported Models"="", "Instrument Options"="", "Flags"=0, "Help"="If ON, the instrument saves the data of a selected waveform on each trigger event. The waveform is saved when the acquisition is complete. During saving, the acquisition stops, and restarts when saving is finished. Thus, the waveform update rate decreases significantly.\n\nAvailable Repeated Capabilities:\nNone\n\nRemote-control command(s):\nTRIGger:EVENt:WFMSave"}, {"Level"=3, "Class Only"=FALSE, "Identifier"="RSRTX_ATTR_ACTIONS_ON_TRIGGER_SAVE_WAVEFORM_DESTINATION", "Descriptive Name"="Actions On Trigger Save Waveform Destination", "Data Type"=2, "Command"="TRIG:EVEN:WFMS:DEST", "Access"=2, "Range Table"="", "Read Callback"="", "Write Callback"="", "Supported Models"="", "Instrument Options"="", "Flags"=0, "Help"="Defines the target directory and file name for a waveform that is saved on trigger event when RSRTX_ATTR_ACTIONS_ON_TRIGGER_SAVE_WAVEFORM is ON.\n\nAvailable Repeated Capabilities:\nNone\n\nRemote-control command(s):\nTRIGger:EVENt:WFMSave:DESTination"}, {"Level"=3, "Class Only"=FALSE, "Identifier"="RSRTX_ATTR_ACTIONS_ON_TRIGGER_REFERENCES", "Descriptive Name"="Actions On Trigger References", "Data Type"=3, "Command"="TRIG:EVEN:REFS", "Access"=2, "Range Table"="", "Read Callback"="", "Write Callback"="", "Supported Models"="", "Instrument Options"="", "Flags"=0, "Help"="Saves 
